vi "Microgear_onConnected.vi"(9 "lenght":u8, 10 "msg":string, 11 "topic":string) -> ()   [LabVIEW 2014]
uses:
  QwaveSys_ESP8266/QwaveSys_ESP8266.lvlib
  QwaveSys_Microgear.lvlib
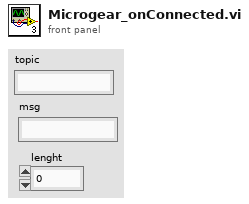
[diagram p1: front panel]
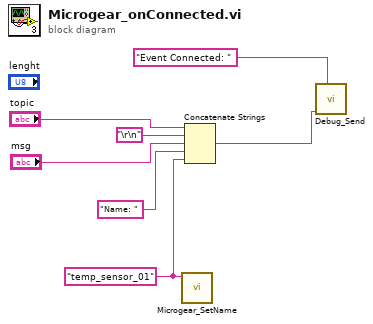
[diagram p0: block diagram]
diagram:
  w1 = "temp_sensor_01" ("name")
  n1 = call "Microgear_SetName.vi"("name"=w1) -> ()  [unwired: 10 in, 1 out]
  n2 = Concatenate Strings("topic", "\r\n" ("End of Line Constant"), "msg", "Name: " ("string"), w1) -> (w2:string)
  n3 = call "Debug_Send.vi"("Name"="Event Connected: ", "DATA"=w2) -> ()  [unwired: 10 in]
